vi "Get Configured Data Channels.vi"(8 "error in (no error)":errorcluster, 10 "framework configuration":T2, 11 "VeriStand Data Sharing Framework in":refnum<class "VeriStand DSF.lvclass">) -> (0 "error out":errorcluster, 1 "data channels refs":T1[](array[typedef]) format="%.0x", 2 "data channel offsets":u64[](array[numeric]) format="%.0x", 3 "VeriStand Data Sharing Framework out":refnum<class "VeriStand DSF.lvclass">)   [LabVIEW 2017, in "DSF Engine.lvlib" / "VeriStand DSF.lvclass"]
uses:
  VeriStand DSF.lvclass
  DSF Core.lvlibp/Typedefs/DSF Engine Framework Configuration.ctl
  DSF Core.lvlibp/Typedefs/DSF Engine Plugin Configuration.ctl
  DSF Core.lvlibp/Typedefs/DSF Timing Info.ctl
  DSF Core.lvlibp/Typedefs/DSF Engine Plugin Thread Configuration.ctl
  DSF Core.lvlibp/Typedefs/DSF Settings Info.ctl
  DSF Core.lvlibp/Typedefs/DSF Engine Transfer Group Configuration.ctl
  DSF Core.lvlibp/Typedefs/DSF Direction.ctl
  DSF Core.lvlibp/Typedefs/DSF Engine Transfer Configuration.ctl
  DSF Core.lvlibp/Typedefs/DSF Byte Order.ctl
  DSF Core.lvlibp/Typedefs/DSF Engine Channel Configuration.ctl
  DSF Core.lvlibp/Typedefs/DSF Data Type.ctl
  DSF Core.lvlibp/Typedefs/DSF Timeout Behavior.ctl
  <vilib>/NI Veristand/Custom Device API/Custom Device Item Ref.ctl
  VeriStand DSF.lvclass/VeriStand DSF.ctl
  <vilib>/NI Veristand/Custom Device API/Data Access Type.ctl
  DSF Core.lvlibp/Classes/Configuration/Channel Count (Transfer).vi
  <vilib>/NI Veristand/Custom Device API/Custom Device API.lvlib
  DSF Core.lvlibp
  DSF Core.lvlibp/Classes/Configuration/Configuration Session.lvclass
  Shared/DSF Shared.lvlib
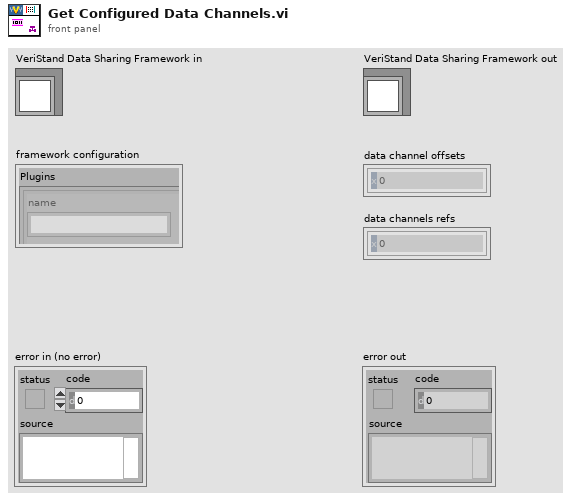
[diagram p1: front panel]
types:
  T1 = typedef "Custom Device API.lvlib/Custom Device Item Ref.ctl" = u64
  T2 = typedef "DSF Core.lvlibp/DSF Engine Framework Configuration.ctl" = cluster{"Plugins":T3[]}
  T3 = typedef "DSF Core.lvlibp/DSF Engine Plugin Configuration.ctl" = cluster{"name":string, "components":string[], "cycle timing":T4, "threads":T5[], "Transfer Groups":T7[], "settings":T6}
  T4 = typedef "DSF Core.lvlibp/DSF Timing Info.ctl" = cluster{"priority":u64, "decimation":u64, "offset":u64}
  T5 = typedef "DSF Core.lvlibp/DSF Engine Plugin Thread Configuration.ctl" = cluster{"buffer converter settings":T6, "transceiver settings":T6, "custom settings":T6, "processor":i32, "priority offset":i16}
  T6 = typedef "DSF Core.lvlibp/DSF Settings Info.ctl" = cluster{"key":string, "value":string}[]
  T7 = typedef "DSF Core.lvlibp/DSF Engine Transfer Group Configuration.ctl" = cluster{"name":string, "direction":T8, "cycle timing":T4, "thread index":i32, "settings":T6, "Transfers":T9[], "timeout behavior":T13}
  T8 = typedef "DSF Core.lvlibp/DSF Direction.ctl" = enum8{"Tx", "Rx"}
  T9 = typedef "DSF Core.lvlibp/DSF Engine Transfer Configuration.ctl" = cluster{"name":string, "byte order":T10, "settings":T6, "channels":T11[]}
  T10 = typedef "DSF Core.lvlibp/DSF Byte Order.ctl" = enum8{"big-endian", "little-endian"}
  T11 = typedef "DSF Core.lvlibp/DSF Engine Channel Configuration.ctl" = cluster{"string offset":u64, "string data type":T12, "engine data type":T12, "name":string, "settings":T6, "units":string}
  T12 = typedef "DSF Core.lvlibp/DSF Data Type.ctl" = enum8{"Bool", "SGL", "DBL", "I8", "I16", "I32", "I64", "U8", "U16", "U32", "U64"}
  T13 = typedef "DSF Core.lvlibp/DSF Timeout Behavior.ctl" = enum8{"Increment Late Count", "Throw Error"}
  T14 = typedef "Custom Device API.lvlib/Data Access Type.ctl" = enum16{"Read", "Write"}
  T15 = typedef "Custom Device API.lvlib/Data Reference.ctl" = i32
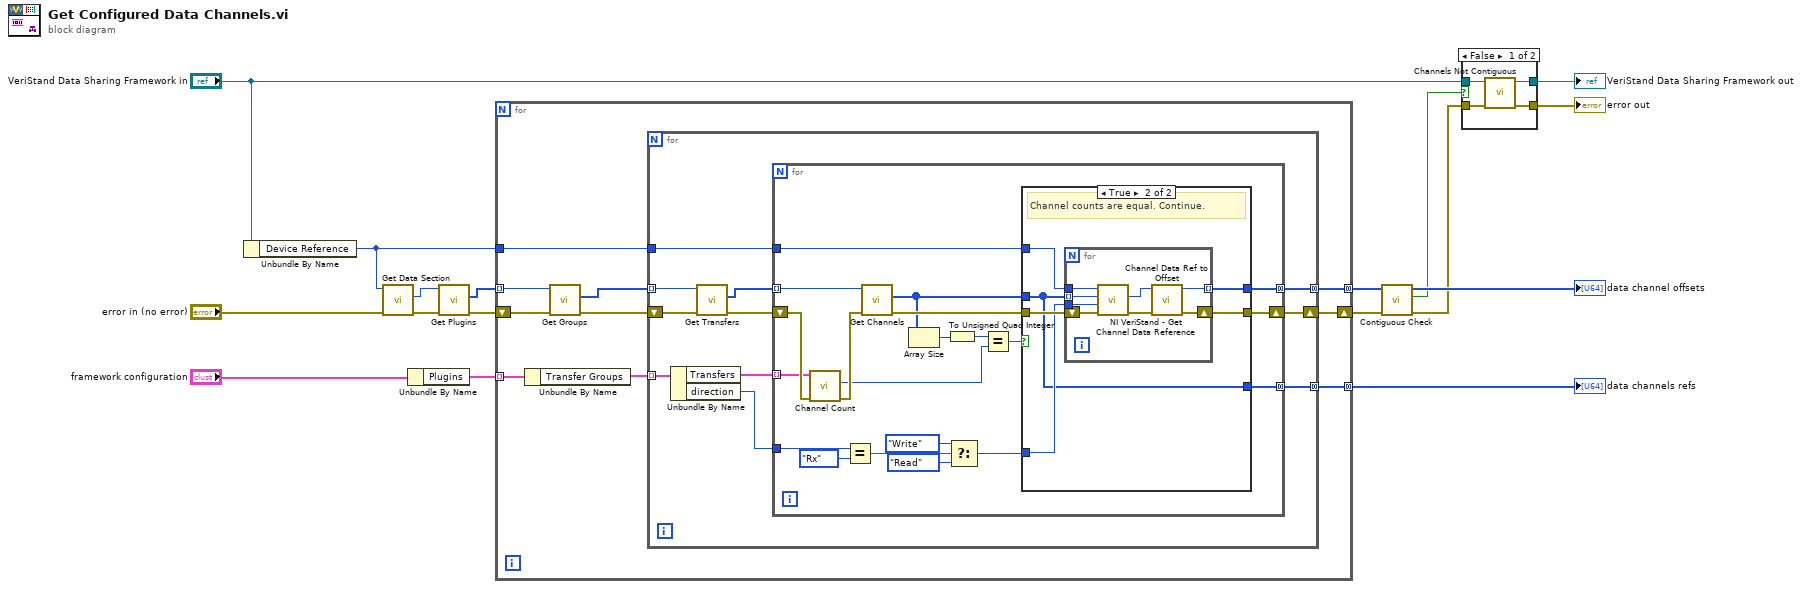
[diagram p0: block diagram]
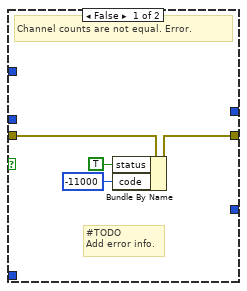
[diagram p2: hidden frame]
diagram:
  n1 = Unbundle By Name("VeriStand Data Sharing Framework in") -> ("Device Reference"=w8:T1)
  n2 = call "Get Data Section.vi"("error in (no error)"="error in (no error)", "Item Ref in"=w8) -> ("error out"=w10:errorcluster, "Data Section ref"=w9:T1)  [unwired: 6 in, 2 out]
  n3 = Unbundle By Name("framework configuration") -> ("Plugins"=w17:T3[])
  n4 = call "Get Plugins.vi"("error in (no error)"=w10, "Item Ref in"=w9) -> ("error out"=w14:errorcluster, "Plugin refs"=w13:T1[])  [unwired: 7 in, 1 out]
  n5 = for {
    tunnel: w13 -> [w21] mode=indexing
    tunnel: w17 -> [w27] mode=indexing
    tunnel: w8 -> [w26]
    shift-right: [w25] -> w15
    shift-left: w14 -> [w22]
    tunnel: [w24] -> w12 mode=concatenating
    tunnel: [w18] -> w1 mode=concatenating
    n6 = Unbundle By Name(w27) -> ("Transfer Groups"=w23:T7[])
    n7 = call "Get Groups.vi"("error in (no error)"=w22, "Plugin Ref in"=w21) -> ("error out"=w20:errorcluster, "Group refs"=w19:T1[])  [unwired: 7 in, 1 out]
    n8 = for {
      tunnel: w23 -> [w38] mode=indexing
      tunnel: w19 -> [w31] mode=indexing
      tunnel: w26 -> [w37]
      shift-right: [w36] -> w25
      shift-left: w20 -> [w32]
      tunnel: [w35] -> w24 mode=concatenating
      tunnel: [w28] -> w18 mode=concatenating
      n9 = Unbundle By Name(w38) -> ("Transfers"=w34:T9[], "direction"=w33:T8)
      n10 = call "Get Transfers.vi"("error in (no error)"=w32, "Group Ref in"=w31) -> ("error out"=w30:errorcluster, "Transfer refs"=w29:T1[])  [unwired: 7 in, 1 out]
      n11 = for {
        tunnel: w34 -> [w47] mode=indexing
        tunnel: w29 -> [w43] mode=indexing
        tunnel: w33 -> [w57]
        tunnel: w37 -> [w50]
        shift-right: [w46] -> w36
        shift-left: w30 -> [w48]
        tunnel: [w45] -> w35 mode=concatenating
        tunnel: [w39] -> w28 mode=concatenating
        n12 = call-poly "Channel Count.vi"("error in (no error)"=w48, "Transfer Configuration in"=w47) -> ("error out"=w44:errorcluster, "total channel count"=w40:u64)  [unwired: 7 in, 1 out]
        n13 = Equal?(x=w57, y=DSF_Direction."Rx") -> (x = y?=w55:bool)
        n14 = call "Get Channels.vi"("error in (no error)"=w44, "Item Ref in"=w43) -> ("error out"=w42:errorcluster, "Channels refs"=w41:T1[])  [unwired: 7 in, 1 out]
        n15 = Array Size(array=w41) -> (size(s)=w58:i32)
        n16 = To Unsigned Quad Integer(1:w58) -> (0:w51:u64)
        n17 = Select(t=Data_Access_Type."Write" ("Access"), s=w55, f=Data_Access_Type."Read") -> (s? t:f=w49:T14)
        n18 = Equal?(x=w51, y=w40) -> (x = y?=w52:bool)
        n19 = case shown="True" w52 {
          tunnel: w41 -> [_ w63]
          tunnel: w50 -> [_ w67]
          tunnel: w49 -> [_ w66]
          tunnel: w42 -> [w62 w68]
          tunnel: [w61 w64] -> w46
          tunnel: [_ w65] -> w45
          tunnel: [_ w63] -> w39
          frame False {
            # "#TODO\nAdd error info."
            # "Channel counts are not equal. Error."
            n20 = Bundle By Name(cluster=w62, "status"=TRUE, "code"=-11000) -> (w61:errorcluster)
          }
          frame True {
            # "Channel counts are equal. Continue."
            n21 = for {
              tunnel: w67 -> [w75]
              tunnel: w66 -> [w74]
              tunnel: w63 -> [w73] mode=indexing
              tunnel: [w69] -> w65 mode=indexing
              shift-right: [w70] -> w64
              shift-left: w68 -> [w76]
              n22 = call <vilib>:"NI VeriStand - Get Channel Data Reference.vi"("error in (no error)"=w76, "Access"=w74, "Channel Ref in"=w73, "Device Ref in"=w75) -> ("error out"=w72:errorcluster, "Channel Data Reference"=w71:T15)  [unwired: 5 in, 1 out]
              n23 = call "Channel Data Ref to Offset.vi"("error in (no error)"=w72, "Channel Data Reference"=w71) -> ("error out"=w70:errorcluster, "channel offset"=w69:u64)  [unwired: 8 in]
            }
          }
        }
      }
    }
  }
  "data channels refs" <- w1
  n24 = call "Contiguous Check.vi"("error in (no error)"=w15, "channel offsets in"=w12) -> ("error out"=w4:errorcluster, "contiguous?"=w2:bool, "channel offsets out"=→"data channel offsets":u64[])  [unwired: 7 in]
  n25 = case shown="False" w2 {
    tunnel: "VeriStand Data Sharing Framework in" -> [w80 w82]
    tunnel: [w79 w82] -> w5
    tunnel: [w78 w81] -> w3
    tunnel: w4 -> [w77 w81]
    frame False {
      n26 = call "Channels Not Contiguous.vi"("error in (no error)"=w77, "VeriStand DSF in"=w80) -> ("error out"=w78:errorcluster, "VeriStand DSF out"=w79:refnum<class "VeriStand DSF.lvclass">)  [unwired: 8 in]
    }
    frame True {
    }
  }
  "error out" <- w3
  "VeriStand Data Sharing Framework out" <- w5
